vi "Parse Named Column as JSON Array.vi"(7 "SpreadsheetDocument in":refnum<k24>, 8 "error in":errorcluster, 9 "Cells":variant[](array[variant]), 10 "Named Range":string, 11 "<JSON>":string="{}") -> (0 "error out":errorcluster, 3 "<JSON> out":string)   [LabVIEW 2025, in "Config from Excel Table.lvclass"]
uses:
  Config from Excel Table.lvclass
  <vilib>/Peter/Open Xml/Source/DocumentFormat.OpenXml.dll
  3d530874-43db-4d28-b45c-a44206ee6d76.vi
  <vilib>/JDP Science/JSONtext/Next JSON Value.vi
  <vilib>/JDP Science/JSONtext/String Subset.vi
  <vilib>/JDP Science/JSONtext/Parsing/Advance past next JSON Value (inlined COPY).vi
  <vilib>/JDP Science/JSONtext/Parsing/Advance past whitespace.vi
  <vilib>/JDP Science/JSONtext/Parsing/Advance past String.vi
  <vilib>/JDP Science/JSONtext/Parsing/Advance past Number.vi
  <vilib>/JDP Science/JSONtext/Parsing/Advance past Line Ending.vi
  <vilib>/JDP Science/JSONtext/Parsing/Parse Full Path or Item Name.vi
  <vilib>/JDP Science/JSONtext/Parsing/Advance past Array.vi
  <vilib>/JDP Science/JSONtext/Parsing/Advance past Object.vi
  <vilib>/JDP Science/JSONtext/support/Error Cluster From Code.vi
  <vilib>/JDP Science/JSONtext/Offset/Find Item Locations by Path.vi
  <vilib>/JDP Science/JSONtext/Variant to JSON Text.vi
  <vilib>/JDP Science/JSONtext/support/Format JSON Array Text.vi
  <vilib>/JDP Science/JSONtext/LVClass Serializer/JSONtext LVClass Serializer.lvclass
  Config from Excel Table.lvclass/Config from Excel Table.ctl
  <vilib>/JDP Science/JSONtext/JSONtext.lvlib
  <vilib>/Peter/Open Xml/Source/Open Xml.lvlib
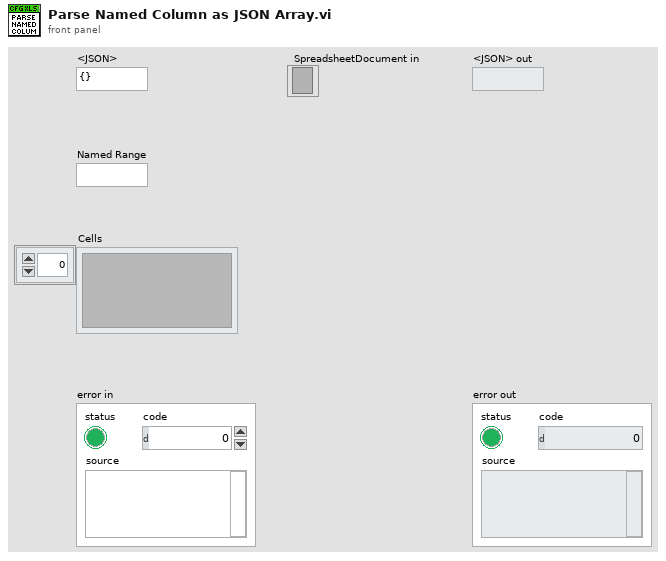
[diagram p1: front panel]
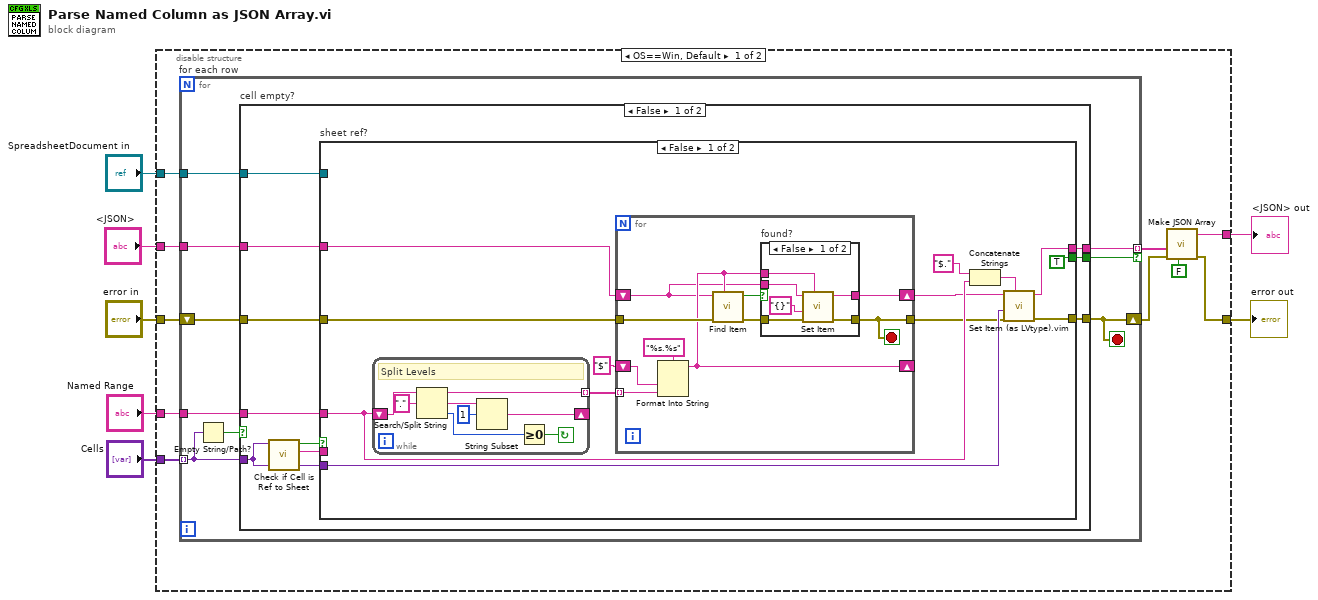
[diagram p0: block diagram]
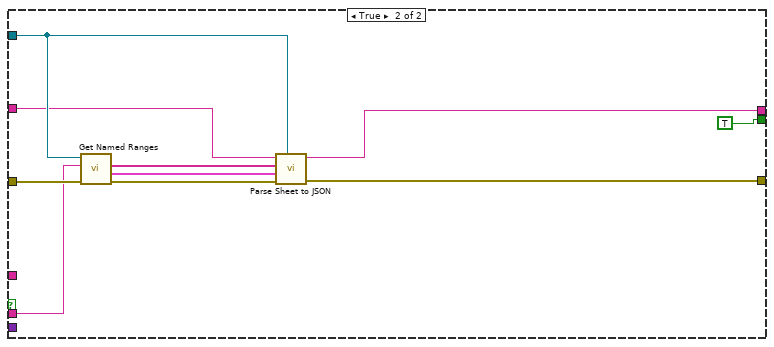
[diagram p3: hidden frame]
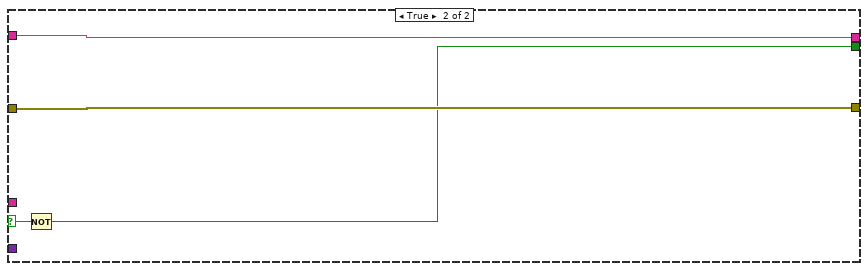
[diagram p4: hidden frame]
diagram:
  n1 = disable-structure shown="OS==Win, Default" {
    disable-tunnel: "Named Range" -> [w17 _]
    disable-tunnel: "<JSON>" -> [w16 _]
    disable-tunnel: "error in" -> [w15 w90]
    disable-tunnel: "SpreadsheetDocument in" -> [w14 _]
    disable-tunnel: "Cells" -> [w13 _]
    disable-tunnel: [w10 _] -> w2
    disable-tunnel: [w8 w90] -> w1
    frame condition #0 (active) {
      n2 = for "for each row" {
        tunnel: w13 -> [w19] mode=indexing
        tunnel: w14 -> [w25]
        shift-right: [w21] -> w9
        shift-left: w15 -> [w26]
        tunnel: w17 -> [w23]
        tunnel: w16 -> [w24]
        tunnel: [w22] -> w12 mode=indexing if=w20
        stop <- w21 stop-if-true
        n3 = Empty String/Path?(string/path=w19) -> (empty?=w18:bool)
        n4 = case "cell empty?" shown="False" w18 {
          selector: w18 -> [_ w87]
          tunnel: w26 -> [w36 w89]
          tunnel: w25 -> [w35 _]
          tunnel: w19 -> [w32 _]
          tunnel: w24 -> [w31 w88]
          tunnel: w23 -> [w30 _]
          tunnel: [w29 w89] -> w21
          tunnel: [w28 w88] -> w22
          tunnel: [w27 w86] -> w20
          frame False {
            n5 = call "Check if Cell is Ref to Sheet.vi"("Value"=w32) -> ("Sheet Name"=w34:string, "Sheet Ref"=w33:bool)  [unwired: 9 in]
            n6 = case "sheet ref?" shown="False" w33 {
              tunnel: w36 -> [w41 w85]
              tunnel: w35 -> [_ w78]
              tunnel: w34 -> [_ w84]
              tunnel: [w45 w82] -> w29
              tunnel: w32 -> [w47 _]
              tunnel: w31 -> [w38 w77]
              tunnel: w30 -> [w44 _]
              tunnel: [w46 w81] -> w28
              tunnel: [TRUE TRUE] -> w27
              frame False {
                n7 = while {
                  shift-right: [w70] -> _
                  shift-left: w44 -> [w69]
                  tunnel: [w68] -> w43 mode=indexing
                  stop <- w71 continue-if-true
                  # "Split Levels"
                  n8 = Search/Split String(string=w69, search string/char (-)=".") -> (substring before match=w68:string, match + rest of string=w72:string, offset of match=w74:i32)  [unwired: 1 in]
                  n9 = String Subset(string=w72, offset (0)=1) -> (substring=w70:string)  [unwired: 1 in]
                  n10 = Greater Or Equal To 0?(x=w74) -> (x >= 0?=w71:bool)
                }
                n11 = for {
                  tunnel: w43 -> [w57] mode=indexing
                  shift-right: [w52] -> _
                  shift-left: "$" -> [w58]
                  tunnel: w41 -> [w55]
                  tunnel: [w54] -> w40
                  shift-right: [w51] -> w39
                  shift-left: w38 -> [w50]
                  stop <- w54 stop-if-true
                  n12 = Format Into String(format string="%s.%s", w58, w57) -> (resulting string=w52:string)  [unwired: 2 in, 1 out]
                  n13 = call <vilib>:"Find Item.vi"("$Path or Item Name"=w52, "error in (no error)"=w55, "JSON"=w50) -> ("error out"=w56:errorcluster, "Found"=w53:bool)  [unwired: 5 in, 2 out]
                  n14 = case "found?" shown="False" w53 {
                    tunnel: [w64 w66] -> w51
                    tunnel: [w63 w67] -> w54
                    tunnel: w56 -> [w62 w67]
                    tunnel: w52 -> [w61 _]
                    tunnel: w50 -> [w60 w66]
                    frame False {
                      n15 = call <vilib>:"Set Item.vi"("$Path or Item Name"=w61, "error in (no error)"=w62, "JSON to Insert"="{}", "JSON"=w60) -> ("error out"=w63:errorcluster, "<JSON>"=w64:string)  [unwired: 4 in, 1 out]
                    }
                    frame True {
                    }
                  }
                }
                n16 = Concatenate Strings("$." ("string"), w44) -> (w48:string)
                n17 = call "Set Item (as LVtype).vim"("$Path or Item Name"=w48, "error in (no error)"=w40, "Anything"=w47, "JSON"=w39) -> ("error out"=w45:errorcluster, "<JSON>"=w46:string)  [unwired: 4 in, 1 out]
              }
              frame True {
                n18 = call <vilib>:"Get Named Ranges.vi"("error in"=w85, "Sheet Name"=w84, "SpreadsheetDoc in"=w78) -> ("error out"=w83:errorcluster, "Cells"=w80:cluster{"Cells":variant[][]}[], "Range Names"=w79:string[])  [unwired: 5 in, 1 out]
                n19 = call "Parse Sheet to JSON.vi"("SpreadsheetDocument in"=w78, "error in"=w83, "Cells"=w80, "Named Ranges"=w79, "<JSON> in"=w77) -> ("error out"=w82:errorcluster, "<JSON> out"=w81:string)  [unwired: 5 in]
              }
            }
          }
          frame True {
            n20 = Not(x=w87) -> (.not. x?=w86:bool)
          }
        }
      }
      n21 = call <vilib>:"Make JSON Array.vi"("Pretty Print?"=FALSE, "error in (no error)"=w9, "JSON Elements"=w12) -> ("error out"=w8:errorcluster, "<JSON>"=w10:string)  [unwired: 7 in]
    }
    frame condition #1 {
    }
  }
  "error out" <- w1
  "<JSON> out" <- w2
